vi "Device Close.vi"(8 "error in (no error)":errorcluster caption="错误输入（无错误）") -> (0 "error out":errorcluster caption="错误输出")   [LabVIEW 2018, in "CAN FD.lvlib"]
uses:
  CAN FD.lvlib
  SubVI/zlgcan.lvlib
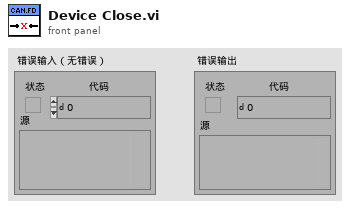
[diagram p1: front panel]
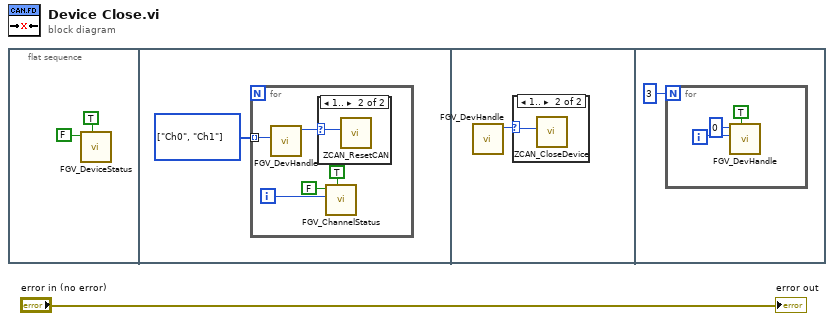
[diagram p0: block diagram]
diagram:
  n1 = flat-sequence {
    frame #0 {
      n2 = call "FGV_DeviceStatus.vi"("Set"=TRUE, "Open"=FALSE) -> ()  [unwired: 8 in, 2 out]
    }
    frame #1 {
      w4 = enum16{"Device", "Ch0", "Ch1"}[] [enum."Ch0", enum."Ch1"] items=["Device", "Ch0", "Ch1"]
      n3 = for {
        tunnel: w4 -> [w9] mode=indexing
        i -> [w7]
        n4 = call "FGV_DevHandle.vi"("Type"=w9) -> ("handle out"=w8:u64)  [unwired: 8 in, 2 out]
        n5 = case shown="1.." w8 {
          selector: w8 -> [_ w10]
          frame 0 {
          }
          frame 1.. {
            n6 = call "ZCAN_ResetCAN.vi"("can_handle"=w10) -> ()  [unwired: 9 in, 2 out]
          }
        }
        n7 = call "FGV_ChannelStatus.vi"("Set"=TRUE, "Index"=w7, "Start"=FALSE) -> ()  [unwired: 7 in, 2 out]
      }
    }
    frame #2 {
      n8 = call "FGV_DevHandle.vi"() -> ("handle out"=w11:u64)  [unwired: 9 in, 2 out]
      n9 = case shown="1.." w11 {
        selector: w11 -> [_ w12]
        frame 0 {
        }
        frame 1.. {
          n10 = call "ZCAN_CloseDevice.vi"("device_handle"=w12) -> ()  [unwired: 9 in, 2 out]
        }
      }
    }
    frame #3 {
      n11 = for {
        N: 3 -> [_]
        i -> [w16]
        n12 = call "FGV_DevHandle.vi"("Set"=TRUE, "Type"=w16, "handle"=u64 0) -> ()  [unwired: 6 in, 3 out]
      }
    }
  }
  "error out" <- "error in (no error)"
